vi "FTW-Messenger-Destroy.vi"(0 "Messenger":refnum<class "FTW-Messenger.lvclass">, 11 "error in":errorcluster) -> (15 "error out":errorcluster)   [LabVIEW 2014, in "FTW-Messenger.lvclass"]
uses:
  FTW-Messenger.lvclass
panel:
  # "Inputs"
  # "Outputs"
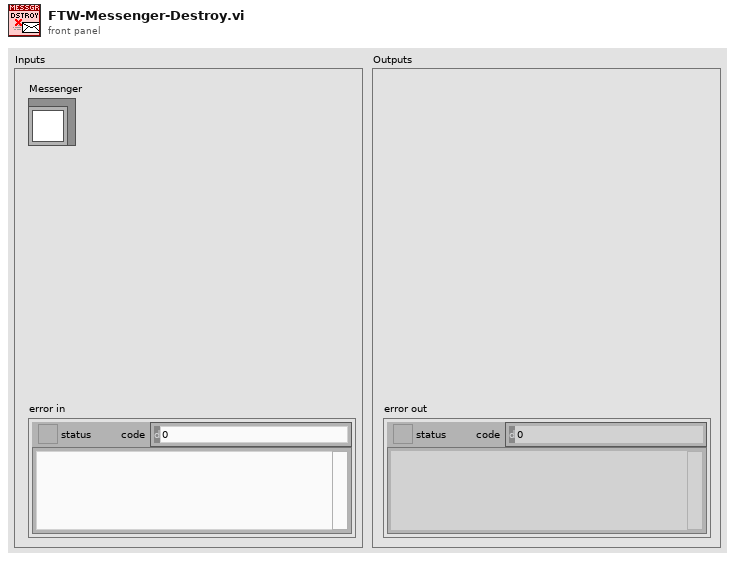
[diagram p1: front panel]
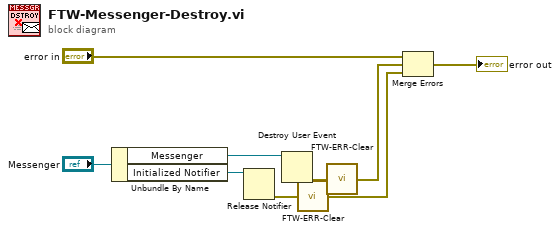
[diagram p0: block diagram]
diagram:
  n1 = Unbundle By Name("Messenger") -> ("Messenger"=w8:refnum<user-event>, "Initialized Notifier"=w2:refnum<notifier>)
  n2 = Release Notifier(notifier=w2) -> (error out=w3:errorcluster)  [unwired: 2 in, 2 out]
  n3 = Destroy User Event(user event=w8) -> (error out=w5:errorcluster)  [unwired: 1 in]
  n4 = call "FTW-ERR-Clear.vi"("error to snuff"=w3) -> ("no error"=w1:errorcluster)
  n5 = call "FTW-ERR-Clear.vi"("error to snuff"=w5) -> ("no error"=w4:errorcluster)
  n6 = Merge Errors("error in", w4, w1) -> (→"error out":errorcluster)
